vi "get_phase_element.vi"(9 "index r":dbl, 10 "hz":dbl, 11 "Array":dbl[][](array[numeric])) -> (3 "element":dbl)   [LabVIEW 2014]
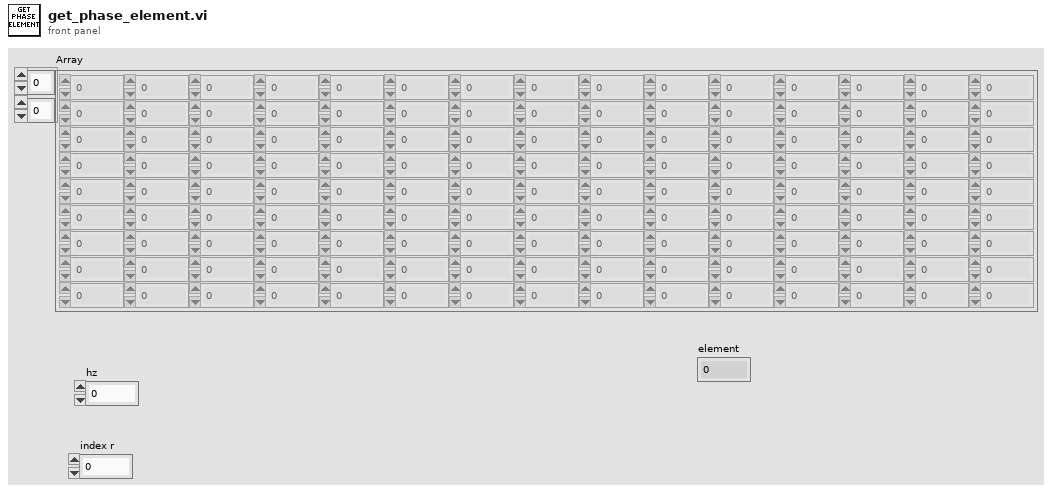
[diagram p1: front panel]
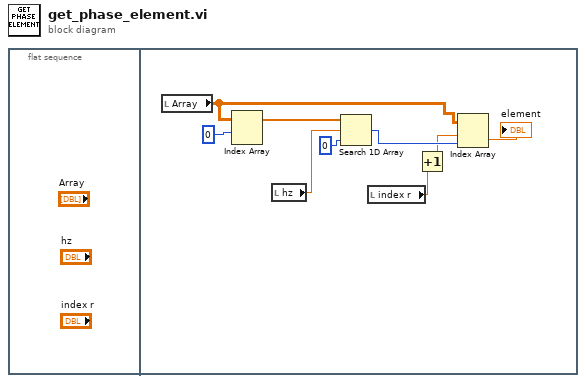
[diagram p0: block diagram]
diagram:
  n1 = flat-sequence {
    frame #0 {
    }
    frame #1 {
      n2 = local read "Array"() -> (w5:dbl[][])
      n3 = Index Array(array=w5, index (row)=0) -> (element=w9:dbl[])  [unwired: 1 in]
      n4 = local read "hz"() -> (w7:dbl)
      n5 = Search 1D Array(1D array=w9, element=w7, start index (0)=0) -> (index of element=w4:i32)
      n6 = local read "index r"() -> (w3:dbl)
      n7 = Increment(x=w3) -> (x+1=w2:dbl)
      n8 = Index Array(array=w5, index (row)=w2, index (col)=w4) -> (element=→"element":dbl)
    }
  }
